vi "Update Finger Kinematics.vi"(8 "error in (no error)":errorcluster, 11 "MF3 in":refnum<class "MF3.lvclass">) -> (0 "error out":errorcluster, 3 "MF3 out":refnum<class "MF3.lvclass">)   [LabVIEW 2013, in "MF3.lvclass"]
uses:
  MF3.lvclass
  MF3.lvclass/MF3.ctl
  Finger/Finger.lvclass
  <vilib>/robotics/Kinematics/NI_Kinematics.lvlib
  <vilib>/ptbypt/NI_PtbyPt.lvlib
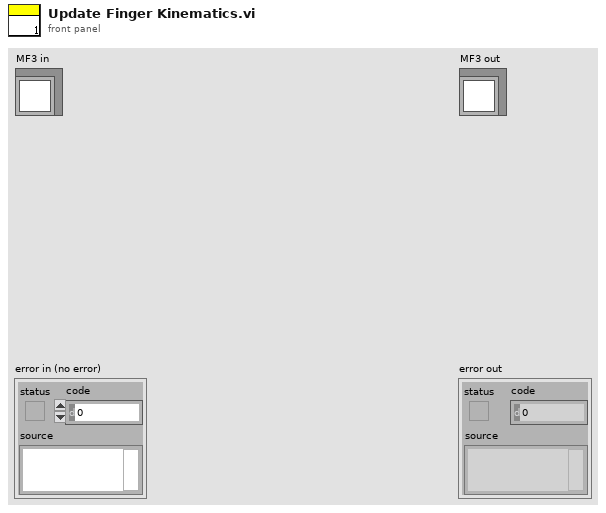
[diagram p1: front panel]
types:
  T1 = typedef "Vector3D Fingers.ctl" = cluster{"Thumb":dbl[], "Middle":dbl[], "Index":dbl[]}
  T2 = typedef "NI_Matrix.lvlib/RealMatrix.ctl" = dbl[][]
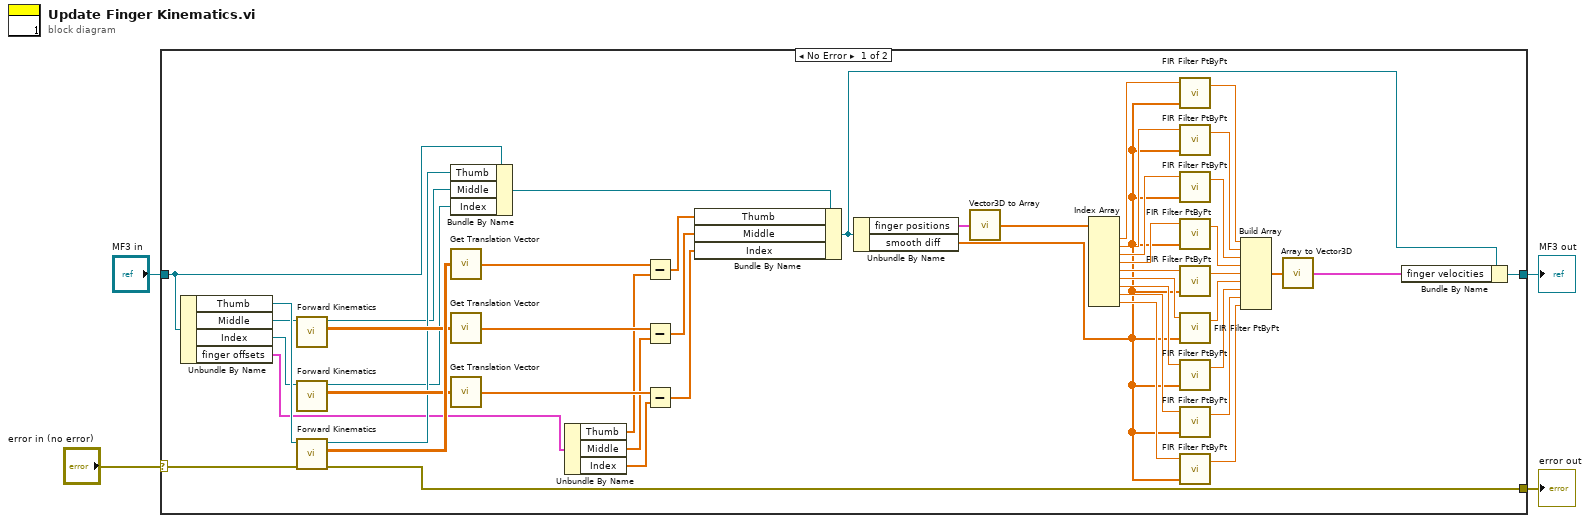
[diagram p0: block diagram]
diagram:
  n1 = case shown="No Error" "error in (no error)" {
    selector: "error in (no error)" -> [w51 w54]
    tunnel: [w50 w54] -> w3
    tunnel: [w26 w53] -> w1
    tunnel: "MF3 in" -> [w44 w53]
    frame No Error {
      n2 = Unbundle By Name(w44) -> ("Thumb"=w52:refnum<class "Finger.lvclass">, "Middle"=w48:refnum<class "Finger.lvclass">, "Index"=w47:refnum<class "Finger.lvclass">, "finger offsets"=w40:T1)
      n3 = call "Forward Kinematics.vi"("Finger in"=w48) -> ("T"=w46:T2, "Finger out"=w42:refnum<class "Finger.lvclass">)  [unwired: 8 in, 1 out]
      n4 = call "Forward Kinematics.vi"("Finger in"=w47) -> ("T"=w45:T2, "Finger out"=w41:refnum<class "Finger.lvclass">)  [unwired: 8 in, 1 out]
      n5 = call "Forward Kinematics.vi"("error in (no error)"=w51, "Finger in"=w52) -> ("error out"=w50:errorcluster, "T"=w49:T2, "Finger out"=w43:refnum<class "Finger.lvclass">)  [unwired: 7 in]
      n6 = Bundle By Name(cluster=w44, "Thumb"=w43, "Middle"=w42, "Index"=w41) -> (w32:refnum<class "MF3.lvclass">)
      n7 = call <vilib>:"Get Translation Vector.vi"("transform"=w49) -> ("translation vector"=w37:dbl[])
      n8 = call <vilib>:"Get Translation Vector.vi"("transform"=w46) -> ("translation vector"=w39:dbl[])
      n9 = call <vilib>:"Get Translation Vector.vi"("transform"=w45) -> ("translation vector"=w38:dbl[])
      n10 = Unbundle By Name(w40) -> ("Thumb"=w34:dbl[], "Middle"=w36:dbl[], "Index"=w35:dbl[])
      n11 = Subtract(x=w37, y=w34) -> (x-y=w31:dbl[])
      n12 = Subtract(x=w39, y=w36) -> (x-y=w30:dbl[])
      n13 = Subtract(x=w38, y=w35) -> (x-y=w33:dbl[])
      n14 = Bundle By Name(cluster=w32, "Thumb"=w31, "Middle"=w30, "Index"=w33) -> (w27:refnum<class "MF3.lvclass">)
      n15 = Unbundle By Name(w27) -> ("finger positions"=w29:T1, "smooth diff"=w5:dbl[])
      n16 = call "Vector3D to Array.vi"("Vector3D"=w29) -> ("Array"=w16:dbl[])
      n17 = Index Array(array=w16) -> (element #1=w15:dbl, element #2=w14:dbl, element #3=w13:dbl, element #4=w12:dbl, element #5=w11:dbl, element #6=w10:dbl, element #7=w9:dbl, element #8=w8:dbl, element #9=w7:dbl)  [unwired: 9 in]
      n18 = call <vilib>:"FIR Filter PtByPt.vi"("Forward Coefficients"=w5, "x"=w15) -> ("Filtered x"=w25:dbl)  [unwired: 2 in, 1 out]
      n19 = call <vilib>:"FIR Filter PtByPt.vi"("Forward Coefficients"=w5, "x"=w14) -> ("Filtered x"=w24:dbl)  [unwired: 2 in, 1 out]
      n20 = call <vilib>:"FIR Filter PtByPt.vi"("Forward Coefficients"=w5, "x"=w13) -> ("Filtered x"=w23:dbl)  [unwired: 2 in, 1 out]
      n21 = call <vilib>:"FIR Filter PtByPt.vi"("Forward Coefficients"=w5, "x"=w12) -> ("Filtered x"=w22:dbl)  [unwired: 2 in, 1 out]
      n22 = call <vilib>:"FIR Filter PtByPt.vi"("Forward Coefficients"=w5, "x"=w11) -> ("Filtered x"=w21:dbl)  [unwired: 2 in, 1 out]
      n23 = call <vilib>:"FIR Filter PtByPt.vi"("Forward Coefficients"=w5, "x"=w10) -> ("Filtered x"=w20:dbl)  [unwired: 2 in, 1 out]
      n24 = call <vilib>:"FIR Filter PtByPt.vi"("Forward Coefficients"=w5, "x"=w9) -> ("Filtered x"=w19:dbl)  [unwired: 2 in, 1 out]
      n25 = call <vilib>:"FIR Filter PtByPt.vi"("Forward Coefficients"=w5, "x"=w8) -> ("Filtered x"=w18:dbl)  [unwired: 2 in, 1 out]
      n26 = call <vilib>:"FIR Filter PtByPt.vi"("Forward Coefficients"=w5, "x"=w7) -> ("Filtered x"=w17:dbl)  [unwired: 2 in, 1 out]
      n27 = Build Array(w25, w24, w23, w22, w21, w20, w19, w18, w17) -> (w6:dbl[])
      n28 = call "Array to Vector3D.vi"("Array"=w6) -> ("Vector3D"=w28:T1)
      n29 = Bundle By Name(cluster=w27, "finger velocities"=w28) -> (w26:refnum<class "MF3.lvclass">)
    }
    frame Error {
    }
  }
  "error out" <- w3
  "MF3 out" <- w1
